vi "gaussian_fit.vi"(7 "Max Itterations":u32=100, 8 "Y Values":dbl[](array[numeric])=[1.0, 1.0, 1.0, 1.0, 3.0, 10.0, 15.0, 32.0, 43.0, 53.0, 52.0, 41.0, 34.0, 12.0, 9.0, 5.0, 2.0, 1.0, 1.0], 9 "X Values":dbl[](array[numeric])=[1.0, 2.0, 3.0, 4.0, 5.0, 6.0, 7.0, 8.0, 9.0, 10.0, 11.0, 12.0, 13.0, 14.0, 15.0, 16.0, 17.0, 18.0, 19.0]) -> (0 "offset":dbl=0.8835487272199344, 1 "Spread (st dev)":dbl=2.2686485457637424, 2 "Center":dbl=10.468826714487445, 3 "Amplitude":dbl=52.79427246119703, 4 "FWHM":dbl=5.342259070694774, 5 "mean square error":dbl=5.342259070694774)   [LabVIEW 2011]
doc: "This VI calculates a 4th order gaussian fit based on input X and Y arrays. The fit equation is:\n\namplitude * exp(-1*(((x-center)/spread)*((x-center)/spread))/2) + offset"
uses:
  <vilib>/gmath/NI_Gmath.lvlib
panel:
  in  "gaussian model description":T1={"model"="a*exp(-1*(((x-b)/c)*((x-b)/c))/2) + d", "Parameters"=["a", "b", "c", "d"], "x"="x"}
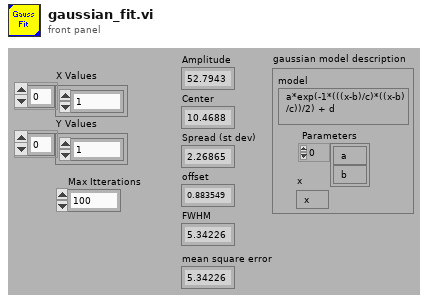
[diagram p1: front panel]
types:
  T1 = cluster{"model":string, "Parameters":string[], "x":string}
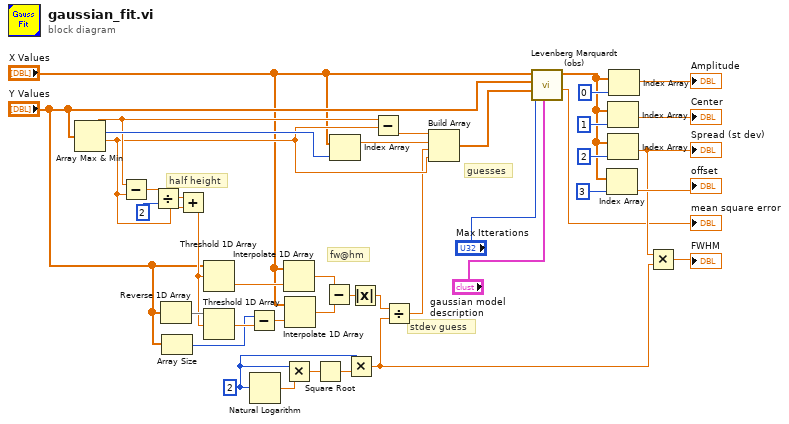
[diagram p0: block diagram]
diagram:
  w26 = 2
  # "guesses"
  # "stdev guess"
  # "fw@hm"
  # "half height"
  n1 = Array Max & Min(array="Y Values") -> (max value=w20:dbl, max index (indices)=w23:i32, min value=w16:dbl)  [unwired: 1 out]
  n2 = Subtract(x=w20, y=w16) -> (x-y=w19:dbl)
  n3 = Divide(x=w19, y=2) -> (x/y=w17:dbl)
  n4 = Reverse 1D Array(array="Y Values") -> (reversed array=w15:dbl[])
  n5 = Array Size(array="Y Values") -> (size(s)=w10:i32)
  n6 = Add(x=w17, y=w16) -> (x+y=w14:dbl)
  n7 = Threshold 1D Array(2:w14, 3:"Y Values") -> (0:w13:dbl)  [unwired: 1 in]
  n8 = Threshold 1D Array(2:w14, 3:w15) -> (0:w11:dbl)  [unwired: 1 in]
  n9 = Subtract(x=w10, y=w11) -> (x-y=w9:dbl)
  n10 = Natural Logarithm(1:w26) -> (0:w29:dbl)
  n11 = Interpolate 1D Array(1:w13, 2:"X Values") -> (0:w7:dbl)
  n12 = Multiply(x=w26, y=w29) -> (x*y=w28:dbl)
  n13 = Interpolate 1D Array(1:w9, 2:"X Values") -> (0:w6:dbl)
  n14 = Square Root(x=w28) -> (sqrt(x)=w27:dbl)
  n15 = Subtract(x=w7, y=w6) -> (x-y=w5:dbl)
  n16 = Index Array(array="X Values", index=w23) -> (element=w22:dbl)
  n17 = Multiply(x=w26, y=w27) -> (x*y=w3:dbl)
  n18 = Absolute Value(x=w5) -> (abs(x)=w4:dbl)
  n19 = Subtract(x=w20, y=w16) -> (x-y=w21:dbl)
  n20 = Divide(x=w4, y=w3) -> (x/y=w2:dbl)
  n21 = Build Array(w21, w22, w2, w16) -> (w36:dbl[])
  n22 = call <vilib>:"Levenberg Marquardt (obs).vi"("model description"="gaussian model description", "max iteration"="Max Itterations", "Initial Guess Coefficient"=w36, "Y"="Y Values", "X"="X Values") -> ("mse"=→"mean square error":dbl, "Best Fit Coefficients"=w31:dbl[])  [unwired: 1 in, 4 out]
  n23 = Index Array(array=w31, index=3) -> (element=→"offset":dbl)
  n24 = Index Array(array=w31, index=1) -> (element=→"Center":dbl)
  n25 = Index Array(array=w31, index=2) -> (element=w24:dbl)
  "Spread (st dev)" <- w24
  n26 = Index Array(array=w31, index=0) -> (element=→"Amplitude":dbl)
  n27 = Multiply(x=w24, y=w3) -> (x*y=→"FWHM":dbl)
